vi "Write.vi"(10 "I32":i32, 11 "I32 in":refnum<class "I32.lvclass">) -> (3 "I32 out":refnum<class "I32.lvclass">)   [LabVIEW 2020, in "Data.lvlib" / "I32.lvclass"]
doc: "Write I32."
uses:
  I32.lvclass
  I32.lvclass/I32.ctl
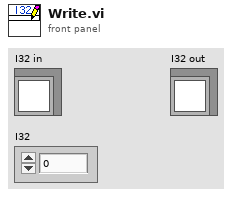
[diagram p1: front panel]
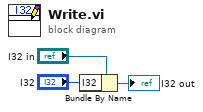
[diagram p0: block diagram]
diagram:
  n1 = Bundle By Name(cluster="I32 in", "I32"="I32") -> (→"I32 out":refnum<class "I32.lvclass">)
